vi "Divide input to 20ms frames.vi"(10 "dt":dbl, 11 "Y":dbl[](array[numeric])) -> (0 "number of columns":i32, 1 "number of rows":i32, 2 "Frames Matrix":dbl[][](array[numeric]), 4 "Frames Array":dbl[](graph))   [LabVIEW 2013]
uses:
  <vilib>/Analysis/4window.llb/Hamming Window (DBL).vi
  <vilib>/Analysis/4window.llb/AllCosWindow (DBL).vi
  <vilib>/Analysis/NI_AALPro.lvlib
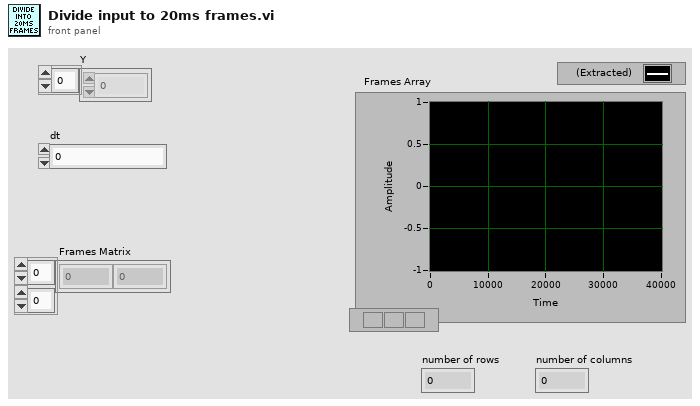
[diagram p1: front panel]
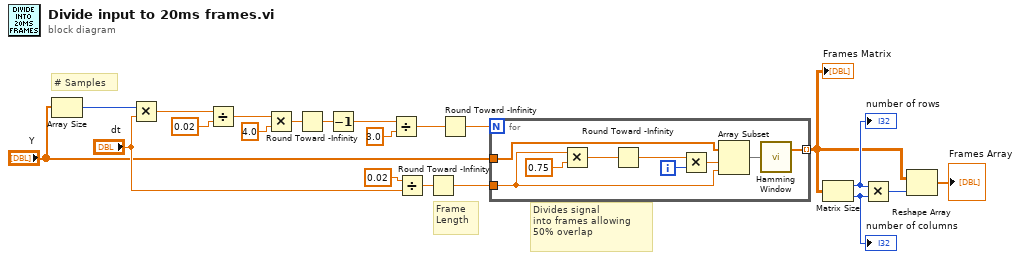
[diagram p0: block diagram]
diagram:
  # "Divides signal \ninto frames allowing \n50% overlap"
  # "Frame \nLength"
  # "# Samples"
  n1 = Array Size(array="Y") -> (size(s)=w21:i32)
  n2 = Multiply(x=w21, y="dt") -> (x*y=w18:dbl)
  n3 = Divide(x=w18, y=0.02) -> (x/y=w14:dbl)
  n4 = Multiply(x=w14, y=4.0) -> (x*y=w13:dbl)
  n5 = Round Toward -Infinity(1:w13) -> (0:w16:dbl)
  n6 = Decrement(x=w16) -> (x-1=w11:dbl)
  n7 = Divide(x=w11, y=3.0) -> (x/y=w10:dbl)
  n8 = Divide(x=0.02, y="dt") -> (x/y=w7:dbl)
  n9 = Round Toward -Infinity(1:w7) -> (0:w8:dbl)
  n10 = Round Toward -Infinity(1:w10) -> (0:w9:dbl)
  n11 = for {
    N: w9 -> [_]
    tunnel: "Y" -> [w30]
    tunnel: w8 -> [w27]
    tunnel: [w22] -> w2 mode=indexing
    i -> [w29]
    n12 = Multiply(x=w27, y=0.75 ("x")) -> (x*y=w25:dbl)
    n13 = Round Toward -Infinity(1:w25) -> (0:w24:dbl)
    n14 = Multiply(x=w24, y=w29) -> (x*y=w26:dbl)
    n15 = Array Subset(array=w30, index=w26, length=w27) -> (w23:dbl[])
    n16 = call-poly <vilib>:"Hamming Window.vi"("X"=w23) -> ("Windowed X"=w22:dbl[])  [unwired: 1 out]
  }
  "Frames Matrix" <- w2
  n17 = Matrix Size(0:w2) -> (1:w6:i32, 2:w5:i32)
  "number of columns" <- w5
  "number of rows" <- w6
  n18 = Multiply(x=w6, y=w5) -> (x*y=w4:i32)
  n19 = Reshape Array(w2, w4) -> (→"Frames Array":dbl[])
